vi "Expt4_MT MSK Transceiver_lab.vi"(0 "# Message Symbols":i32=1000, 7 "Eb/N0, dB":dbl(slide)=40.0 scale=0.0..80.0, 11 "Reset":bool=TRUE, 14 "?":T2(tab)=enum."MSK Constellation (RX)") -> (3 "MSK System Parameters":T5={"Differential Encoding Enable"=enum."enable", "Samples per Symbol (16)"=16}, 4 "Output Complex Waveform":cluster{"t0":dbl, "dt":dbl, "Values":cdb[]} {"Values" format="%.3f"; "dt" format="%^.2e"; "t0" format="%.4f"}, 6 "Transmitted Bits":i8[](array[numeric]), 8 "Received  Bits":i8[](array[numeric]), 10 "Bit Error Rate":dbl format="%.4e", 13 "Last Sync Found Index":dbl format="%.4f", 15 "Error Out":errorcluster)   [LabVIEW 2020]
doc: "This example demonstrates generation and analysis of MSK modulated signals. You can specify transmit filter parameters, Eb/No, and frequency offset. This example demonstrates programming techniques for resetting the transmitter in cases where the receiver (demodulator) lock is lost. You can see the results of the demodulation on trellis graphs, and perform measurements such as bit error rate."
uses:
  <vilib>/addons/Modulation/Digital/Support/Common/Validators/mod_AWGN Validate.vi
  <vilib>/addons/Modulation/Analog/support/mod_Set Error Source.vi
  <vilib>/addons/Modulation/Digital/Impairments/subVIs/mod_createSeeds.vi
  <vilib>/addons/Modulation/Digital/Impairments/subVIs/mod_IQ Impairments Gain Imbalance.vi
  <vilib>/addons/Modulation/Digital/Impairments/subVIs/mod_IQ Impairments Quadrature Skew.vi
  <vilib>/addons/Modulation/Digital/Impairments/subVIs/mod_IQ Impairments Axis Shear.vi
  <vilib>/addons/Modulation/Digital/Impairments/subVIs/mod_IQ Impairments DC Offset.vi
  <vilib>/addons/Modulation/Digital/Impairments/subVIs/mod_IQ Impairments Frequency Offset.vi
  <vilib>/addons/Modulation/Digital/Support/Common/Validators/mod_Validate Samples Per Symbol.vi
  <vilib>/addons/Modulation/Analog/support/Validators/mod_Validate Complex Waveform.vi
  <vilib>/Analysis/5stat.llb/RMS.vi
  <vilib>/Analysis/5stat.llb/RMS (DBL).vi
  <vilib>/addons/Modulation/Digital/Support/Common/mod_Apply Frequency Offset.vi
  <vilib>/addons/Modulation/Analog/support/Validators/mod_WFErrorHandler.vi
  <vilib>/addons/Modulation/Digital/Support/Common/mod_Apply Frequency Offset (Internal).vi
  <vilib>/addons/Modulation/Digital/General/subVIs/mod_Generate Bits PN Sequence.vi
  <vilib>/Analysis/1siggen.llb/Gaussian White Noise (obs 90).vi
  <vilib>/addons/Modulation/Digital/Support/Common/Validators/mod_IQ Impairments Validate.vi
  <vilib>/addons/Modulation/Digital/Demodulation/MT EbN0 Calculation(MSK).vi
  <vilib>/addons/Modulation/Digital/Demodulation/MT Calculate BER After Trigger (PN Sequence).vi
  <vilib>/addons/Modulation/niDMT.lvlib
panel:
  out "Estimated Eb/N0(dB)":dbl
  out "Sampling Rate":dbl format="%.2p"
  in  "BT":dbl=0.5 format="%.2f"
  out "Frequency Offset (Hz)":dbl format="%.2f"
  in  "Frequency Offset (Hz)":dbl(slide) scale=-1000.0..1000.0
  in  "Symbol Rate":dbl=100000.0 step=1000.0 format="%.2p"
  out "Modulation Error Ratio (dB)":dbl format="%.2f"
  out "BER Trigger Found ?":bool
  in  "TX Filter":T1(ring)=enum."Gaussian"
  in  "?":bool
  out "Tx Symbols":T3(graph)={{"1/x"=0.0, 1e-05, [], 1}, []}
  out "TX Constellation":T4(graph)
  out "TX Trellis graph":cluster{dbl, "dt":dbl, dbl[]}[](graph)
  out "RX Symbols":T3(graph)={{"1/x"=0.0, 1e-05, [], 1}, []}
  in  "autoscale":bool
  out "RX Constellation":T4(graph)
  out "RX Trellis Graph":cluster{dbl, "dt":dbl, dbl[]}[](graph)
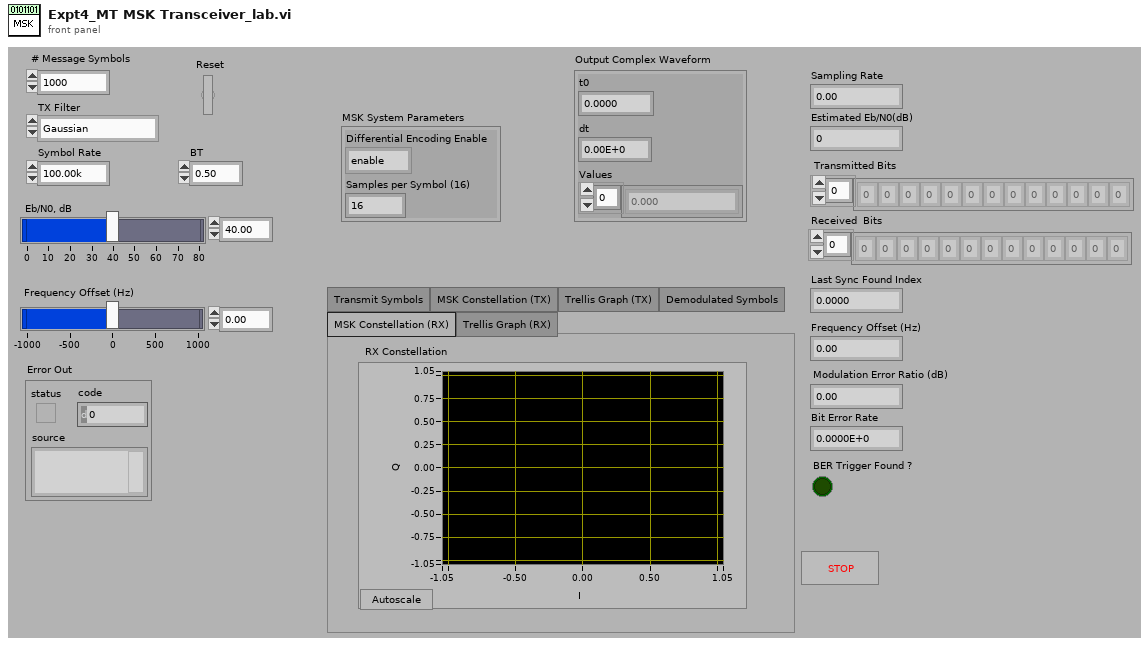
[diagram p1: front panel]
types:
  T1 = enum16{"none", "Raised Cosine", "Root Raised Cos", "Gaussian"}
  T2 = enum32{"Transmit Symbols", "MSK Constellation (TX)", "Trellis Graph (TX)", "Demodulated Symbols", "MSK Constellation (RX)", "Trellis Graph (RX)"}
  T3 = cluster{cluster{"1/x":dbl, dbl, i8[], i32}, i32[][]}
  T4 = cluster{"Decimated Array":dbl[], "Decimated Array":dbl[]}[]
  T5 = cluster{"Differential Encoding Enable":enum16{"disable", "enable"}, "Samples per Symbol (16)":i32}
  T6 = cluster{"expected sync location (symbols)":i32, "sync sequence":cdb[], "sync location uncertainty (symbols)":i32, "sync indent (symbols)":i32}
  T7 = cluster{"TX Filter":enum16{"none", "Raised Cosine", "Root Raised Cos", "Gaussian"}, "filter parameter":dbl, "filter length":i32}
  T8 = cluster{"# Guard Bits":i32, "# Sync Bits":i32, "# Message Bits":i32, "PN sequence order":i32}
  T9 = typedef "niAMT.lvlib/Complex Data Waveform.ctl" = cluster{"t0":dbl, "dt":dbl, "Y":cdb[]}
  T10 = cluster{"Output Bit Stream":i8[], " # bits per symbol":i32, "Sync (Bits)":i8[], "Sync (Symbols)":cdb[], "pulse shaping filter coefficients":dbl[], "matched filter coefficients":dbl[], "MSK system parameters":cluster{"differential encoding enable":enum16{"disable", "enable"}, "samples per symbol (16)":i32}}
  T11 = cluster{"differential encoding enable":enum16{"disable", "enable"}, "samples per symbol (16)":i32}
  T12 = cluster{"frequency offset (Hz)":dbl, "frequency drift (Hz)":dbl}
  T13 = cluster{"constellation":dbl[], "oversampled data":dbl[]}[]
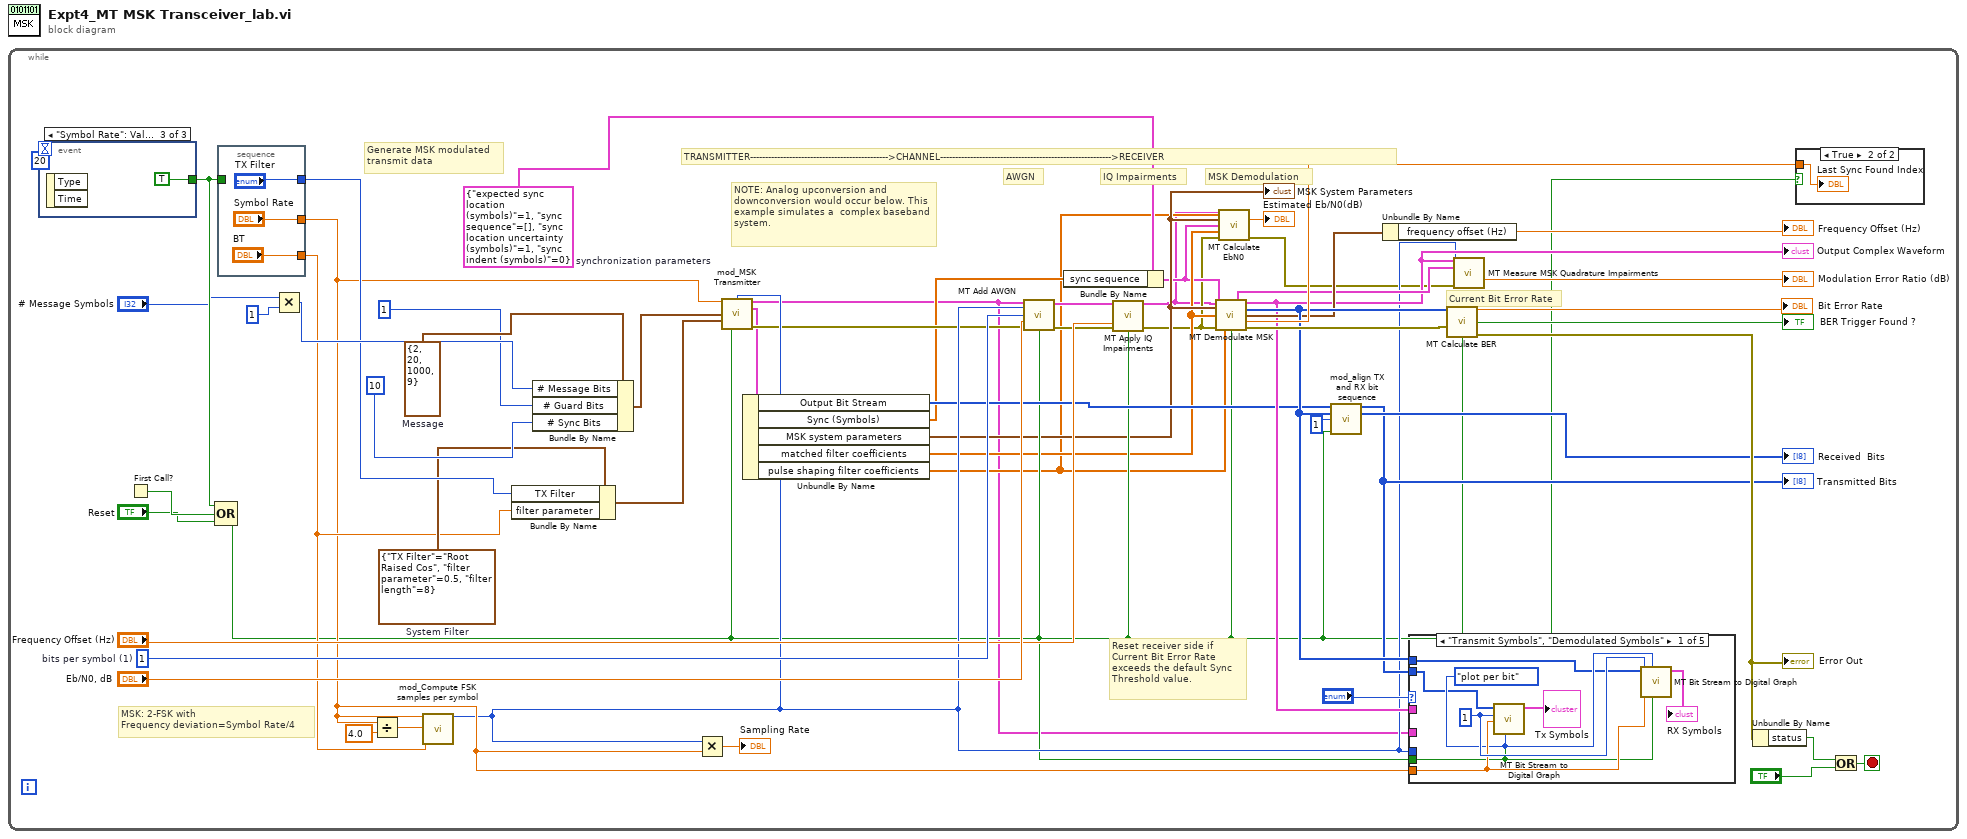
[diagram p0: block diagram]
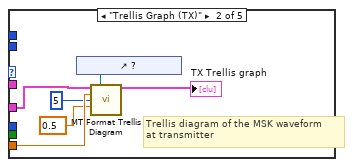
[diagram p2: hidden frame]
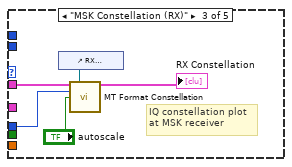
[diagram p3: hidden frame]
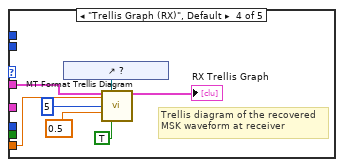
[diagram p4: hidden frame]
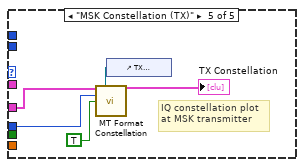
[diagram p5: hidden frame]
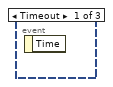
[diagram p7: hidden frame]
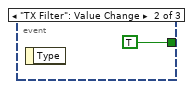
[diagram p8: hidden frame]
diagram:
  n1 = while {
    stop <- w35 stop-if-true
    w18 = T6 {"expected sync location (symbols)"=1, "sync sequence"=[], "sync location uncertainty (symbols)"=1, "sync indent (symbols)"=0}  # synchronization parameters
    w25 = T7 {"TX Filter"=enum."Root Raised Cos", "filter parameter"=0.5, "filter length"=8}  # System Filter
    w39 = 1  # bits per symbol (1)
    w43 = T8 {"# Guard Bits"=2, "# Sync Bits"=20, "# Message Bits"=1000, "PN sequence order"=9}  # Message
    # "IQ Impairments"
    # "NOTE: Analog upconversion and downconversion would occur below. This example simulates a  complex baseband system."
    # "MSK: 2-FSK with\nFrequency deviation=Symbol Rate/4"
    # "Reset receiver side if \nCurrent Bit Error Rate\nexceeds the default Sync \nThreshold value."
    # "AWGN"
    # "Generate MSK modulated\ntransmit data"
    # "MSK Demodulation"
    # "Current Bit Error Rate"
    # "TRANSMITTER---------------------------------------------->CHANNEL--------------------------------------------------------->RECEIVER"
    n2 = event shown="[2] \"Symbol Rate\": Value Change" {
      selector: _ -> [_ _ _]
      dyn-events: _ -> [_ _ _]
      timeout: 20 -> [_ _ _]
      tunnel: [_ TRUE TRUE] -> w48
      event Timeout {
        n3 = event-data() -> ()  [unwired: 1 in, 1 out]
      }
      event "TX Filter": Value Change {
        n4 = event-data() -> ()  [unwired: 1 in, 1 out]
      }
      event "Symbol Rate": Value Change {
        n5 = event-data() -> ()  [unwired: 1 in, 2 out]
      }
    }
    n6 = First Call?() -> (First Call?: T/F=w53:bool)
    n7 = Compound Arithmetic op=OR(w48, w53, "Reset") -> (w11:bool)
    n8 = stacked-sequence {
      tunnel: w48 -> [_]
      tunnel: ["TX Filter"] -> w40
      tunnel: ["Symbol Rate"] -> w20
      tunnel: ["BT"] -> w21
      frame #0 {
      }
    }
    n9 = Multiply(x="# Message Symbols", y=1) -> (x*y=w41:i32)
    n10 = Divide(x=w20, y=4.0) -> (x/y=w23:dbl)
    n11 = call <vilib>:"mod_Compute FSK samples per symbol.vi"("Symbol Rate"=w20, "Deviation (Hz)"=w23, "Filter parameter"=w21) -> ("FSK samples per symbol"=w17:i32)  [unwired: 11 in, 1 out]
    n12 = Bundle By Name(cluster=w25, "TX Filter"=w40, "filter parameter"=w21) -> (w26:T7)
    n13 = Bundle By Name(cluster=w43, "# Message Bits"=w41, "# Guard Bits"=1, "# Sync Bits"=10) -> (w1:T8)
    n14 = Multiply(x=w17, y=w20) -> (x*y=→"Sampling Rate":dbl)
    n15 = call <vilib>:"mod_MSK Transmitter.vi"("Symbol Rate, Hz"=w20, "Reset?"=w11, "# Samples per Symbol"=w17, "Message"=w1, "System Filter"=w26) -> ("Output Complex Waveform"=w2:T9, "Signal Description"=w14:T10, "error out"=w15:errorcluster)  [unwired: 8 in]
    n16 = Unbundle By Name(w14) -> ("Output Bit Stream"=w13:i8[], "Sync (Symbols)"=w12:cdb[], "MSK system parameters"=w10:T11, "matched filter coefficients"=w9:dbl[], "pulse shaping filter coefficients"=w5:dbl[])
    "MSK System Parameters" <- w10
    n17 = call <vilib>:"MT Add AWGN.vi"("input complex waveform"=w2, "samples per symbol (16)"=w17, "bits per symbol (1)"=w39, "Eb/N0 (10 dB)"="Eb/N0, dB", "error in (no error)"=w15, "reset? (T)"=w11) -> ("output complex waveform"=w32:T9, "error out"=w16:errorcluster)  [unwired: 7 in, 1 out]
    n18 = Bundle By Name(cluster=w18, "sync sequence"=w12) -> (w8:T6)
    n19 = call <vilib>:"MT Apply IQ Impairments.vi"("input complex waveform"=w32, "error in (no error)"=w16, "frequency offset (Hz)"="Frequency Offset (Hz)", "reset? (T)"=w11) -> ("output complex waveform"=w3:T9, "error out"=w7:errorcluster)  [unwired: 10 in]
    n20 = call <vilib>:"MT Demodulate MSK.vi"("input complex waveform"=w3, "MSK system parameters"=w10, "matched filter coefficients"=w9, "synchronization parameters"=w8, "error in (no error)"=w7, "pulse shaping filter coefficients"=w5, "reset? (T)"=w11) -> ("detected complex waveform"=w28:cluster{"t0":dbl, "dt":dbl, "Y":cdb[]}, "recovered complex waveform"=w27:T9, "output bit stream"=w38:i8[], "measurements"=w30:T12, "sync found index (symbols)"=w51:dbl, "error out"=w45:errorcluster)  [unwired: 3 in]
    "Output Complex Waveform" <- w27
    "Received  Bits" <- w38
    n21 = call-poly <vilib>:"MT Calculate EbN0.vi"("Recieved waveform"=w3, "pulse shaping filter coefficients"=w5, "MSK system parameters"=w10, "synchronization parameters"=w8, "matched filter coefficients"=w9, "error in (no error)"=w7) -> ("Eb/N0(dB)"=→"Estimated Eb/N0(dB)":dbl, "error out"=w6:errorcluster)  [unwired: 7 in, 1 out]
    n22 = call <vilib>:"mod_align TX and RX bit sequence.vi"("TX Bit Sequence"=w13, "RX Bit Sequence"=w38, "# Bits removed"=1, "Reset"=w11) -> ("Aligned array"=w36:i8[])  [unwired: 11 in]
    "Transmitted Bits" <- w36
    n23 = Unbundle By Name(w30) -> ("frequency offset (Hz)"=→"Frequency Offset (Hz)":dbl)
    n24 = case shown="\"Transmit Symbols\", \"Demodulated Symbols\"" "?" {
      tunnel: w38 -> [w62 _ _ _ _]
      tunnel: w20 -> [w66 w72 _ w84 _]
      tunnel: w27 -> [_ _ w77 w82 _]
      tunnel: w17 -> [_ _ w76 _ w88]
      tunnel: w36 -> [w63 _ _ _ _]
      tunnel: w11 -> [w64 _ _ _ _]
      tunnel: w2 -> [_ w69 _ _ w87]
      frame "Transmit Symbols", "Demodulated Symbols" {
        w65 = enum16{"single plot", "plot per bit"}."plot per bit" ("Format")
        w67 = 1 ("bits per symbol")
        n25 = call <vilib>:"MT Bit Stream to Digital Graph.vi"("Reset (F)"=w64, "Format"=w65, "Symbol Rate (Hz)"=w66, "bits per symbol"=w67, "Bit Stream"=w63) -> ("Digital Waveform Graph"=→"Tx Symbols":T3)  [unwired: 6 in]
        n26 = call <vilib>:"MT Bit Stream to Digital Graph.vi"("Reset (F)"=w64, "Format"=w65, "Symbol Rate (Hz)"=w66, "bits per symbol"=w67, "Bit Stream"=w62) -> ("Digital Waveform Graph"=→"RX Symbols":T3)  [unwired: 6 in]
      }
      frame "Trellis Graph (TX)" {
        # "Trellis diagram of the MSK waveform \nat transmitter"
        n27 = control-ref of="?"() -> (w73:refnum<vi>)
        n28 = call <vilib>:"MT Format Trellis Diagram.vi"("waveform"=w69, "trellis reference"=w73, "symbol rate (Hz)"=w72, "trellis length"=5, "modulation index"=0.5) -> ("trellis diagram"=→"TX Trellis graph":cluster{"t0":dbl, "dt":dbl, "phase":dbl[]}[])  [unwired: 9 in, 1 out]
      }
      frame "MSK Constellation (RX)" {
        # "IQ constellation plot\nat MSK receiver"
        n29 = control-ref of="RX Constellation"() -> (w78:refnum<vi>)
        n30 = call <vilib>:"MT Format Constellation.vi"("waveform"=w77, "constellation reference"=w78, "samples per symbol"=w76, "autoscale"="autoscale") -> ("constellation graph"=→"RX Constellation":T13)  [unwired: 10 in, 1 out]
      }
      frame "Trellis Graph (RX)", Default {
        # "Trellis diagram of the recovered\nMSK waveform at receiver"
        n31 = control-ref of="?"() -> (w85:refnum<vi>)
        n32 = call <vilib>:"MT Format Trellis Diagram.vi"("waveform"=w82, "trellis reference"=w85, "symbol rate (Hz)"=w84, "trellis length"=5, "modulation index"=0.5, "autoscale"=TRUE) -> ("trellis diagram"=→"RX Trellis Graph":cluster{"t0":dbl, "dt":dbl, "phase":dbl[]}[])  [unwired: 8 in, 1 out]
      }
      frame "MSK Constellation (TX)" {
        # "IQ constellation plot\nat MSK transmitter"
        n33 = control-ref of="TX Constellation"() -> (w90:refnum<vi>)
        n34 = call <vilib>:"MT Format Constellation.vi"("waveform"=w87, "constellation reference"=w90, "samples per symbol"=w88, "autoscale"=TRUE) -> ("constellation graph"=→"TX Constellation":T13)  [unwired: 10 in, 1 out]
      }
    }
    n35 = call-poly <vilib>:"MT Calculate BER.vi"("input bit stream"=w38, "error in (no error)"=w45, "reset? (T)"=w11) -> ("BER"=→"Bit Error Rate":dbl, "trigger found?"=→"BER Trigger Found ?":bool, "error out"=w56:errorcluster)  [unwired: 8 in, 2 out]
    "Error Out" <- w56
    n36 = call <vilib>:"MT Measure MSK Quadrature Impairments.vi"("recovered complex waveform"=w27, "samples per symbol (16)"=w17, "detected complex waveform"=w28, "error in (no error)"=w6) -> ("modulation error ratio (dB)"=→"Modulation Error Ratio (dB)":dbl)  [unwired: 4 in, 7 out]
    n37 = Unbundle By Name(w56) -> ("status"=w55:bool)
    n38 = case shown="True" w11 {
      tunnel: w51 -> [_ w92]
      frame False {
      }
      frame True {
        "Last Sync Found Index" <- w92
      }
    }
    n39 = Or(x=w55, y="?") -> (x .or. y?=w35:bool)
  }
